vi "AAL Resample (const to const, complex single-channel).vi"(7 "reset?":bool, 8 "error in (no error)":errorcluster, 9 "config":T1={"new sample period"=0.0, "Timing Jitter"=enum."Interpolation", "first point location"=0.0, "prototype filter"={"h"=[], "Max Decimation"=1000}} {"prototype filter"."h" format="%.2f"; "first point location" format="%.2f"; "new sample period" format="%.2f"}, 10 "anti-aliasing?":bool=TRUE, 11 "X":cdb[](array[numeric]) format="%.2f") -> (0 "error out":errorcluster, 2 "normalized t0":dbl, 3 "Y":cdb[](array[numeric]) format="%.2f")   [LabVIEW 2017, in "NI_AALPro.lvlib"]
uses:
  NI_AALPro.lvlib
  <resource>/lvanlys.dll
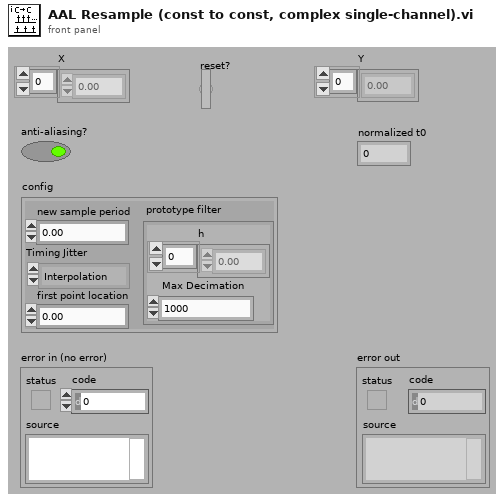
[diagram p1: front panel]
types:
  T1 = cluster{"new sample period":dbl, "Timing Jitter":enum32{"Interpolation", "Rounding"}, "first point location":dbl, "prototype filter":cluster{"h":dbl[], "Max Decimation":i32}}
  T2 = cluster{"precondition":cdb[], "preconditionLen":i32, "extractFilterBuffer":dbl[], "scaling":dbl, "extractFilterLeftLen":i32, "extractFilterRightLen":i32, "method":i32, "new sample period":dbl, "offset":dbl, "index":i32}
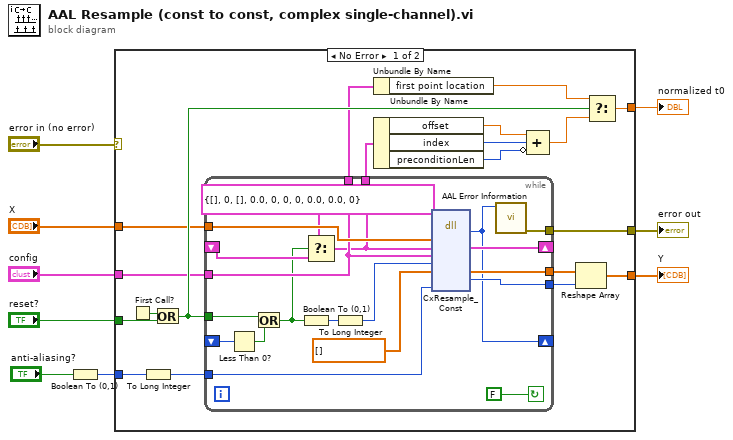
[diagram p0: block diagram]
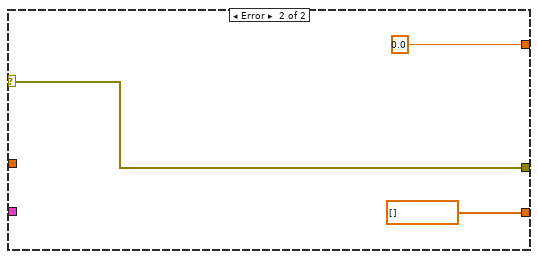
[diagram p2: hidden frame]
diagram:
  n1 = Boolean To (0,1)(Boolean="anti-aliasing?") -> (0, 1=w2:i16)
  n2 = case shown="No Error" "error in (no error)" {
    selector: "error in (no error)" -> [_ w50]
    tunnel: "X" -> [w21 _]
    tunnel: "config" -> [w20 _]
    tunnel: "reset?" -> [w19 _]
    tunnel: [w18 0.0] -> w5
    tunnel: [w17 cdb[] [] ("y")] -> w1
    tunnel: [w16 w50] -> w4
    tunnel: w2 -> [w11 _]
    frame No Error {
      n3 = First Call?() -> (First Call?: T/F=w26:bool)
      n4 = To Long Integer(number=w11) -> (32bit integer=w10:i32)
      n5 = Or(x=w26, y=w19) -> (x .or. y?=w25:bool)
      n6 = while {
        tunnel: w25 -> [w30]
        tunnel: w20 -> [w37]
        tunnel: [w43] -> w27
        tunnel: [w44] -> w28
        shift-left: _ -> [w42]
        shift-right: [w41] -> _
        tunnel: w21 -> [w46]
        tunnel: [w37] -> w24
        tunnel: [w36] -> w23
        tunnel: [w35] -> w16
        tunnel: w10 -> [w34]
        shift-right: [w33] -> _
        shift-left: _ -> [w32]
        stop <- FALSE continue-if-true
        n7 = Less Than 0?(x=w32) -> (x < 0?=w31:bool)
        n8 = Or(x=w30, y=w31) -> (x .or. y?=w29:bool)
        n9 = Boolean To (0,1)(Boolean=w29) -> (0, 1=w39:i16)
        n10 = Select(t=T2 {"precondition"=[], "preconditionLen"=0, "extractFilterBuffer"=[], "scaling"=0.0, "extractFilterLeftLen"=0, "extractFilterRightLen"=0, "method"=0, "new sample period"=0.0, "offset"=0.0, "index"=0} ("state"), s=w29, f=w42) -> (s? t:f=w36:T2)
        n11 = To Long Integer(number=w39) -> (32bit integer=w38:i32)
        n12 = dll-call lib="C:/Program Files (x86)/National Instruments/LabVIEW 2017/resource/lvanlys.*" fn="CxResample_Const"("X"=w46, "state"=w36, "config"=w37, "reset"=w38, "y"=cdb[] [], "bandLimiting"=w34) -> (w33:i32, "state"=w41:T2, "y"=w44:cdb[], "out_len"=w43:i32)  [unwired: 8 in, 2 out]
        n13 = call "AAL Error Information.vi"("error code"=w33) -> ("error out"=w35:errorcluster)  [unwired: 10 in]
      }
      n14 = Unbundle By Name(w24) -> ("first point location"=w22:dbl)
      n15 = Unbundle By Name(w23) -> ("offset"=w12:dbl, "index"=w15:i32, "preconditionLen"=w14:i32)
      n16 = Compound Arithmetic op=ADD(w12, w15, invert w14) -> (w13:dbl)
      n17 = Reshape Array(w28, w27) -> (w17:cdb[])
      n18 = Select(t=w22, s=w25, f=w13) -> (s? t:f=w18:dbl)
    }
    frame Error {
    }
  }
  "error out" <- w4
  "normalized t0" <- w5
  "Y" <- w1
